vi "CloseFile.vi"(8 "error in (no error)":errorcluster, 11 "ReadWrite in":refnum<class "ReadWrite.lvclass">) -> (0 "error out":errorcluster)   [LabVIEW 2021]
uses:
  Interfaces/ReadWrite/ReadWrite.lvclass
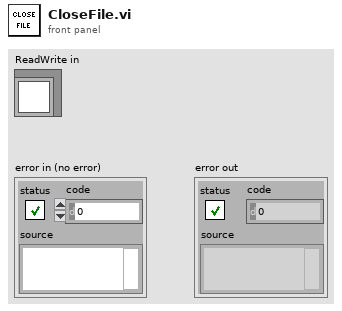
[diagram p1: front panel]
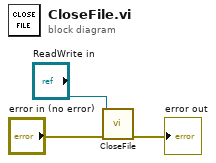
[diagram p0: block diagram]
diagram:
  n1 = call-dynamic "CloseFile.vi"("error in (no error)"="error in (no error)", "ReadWrite in"="ReadWrite in") -> ("error out"=→"error out":errorcluster)  [unwired: 9 in]
